vi "Update Component ID.vi"(8 "error in (no error)":errorcluster, 11 "SMO in":refnum<class "SMO.lvclass">) -> (0 "error out":errorcluster, 3 "SMO out":refnum<class "SMO.lvclass">)   [LabVIEW 2013, in "SMO.lvclass"]
uses:
  SMO.lvclass
  Support/Attribute.Identity/Attribute.Identity.lvclass
  Support/Attribute.Identity/Attribute.Identity.lvclass/Attribute.Identity.ctl
  Support/Attribute.Identity/Calculate Component ID.vi
  <vilib>/Utility/MD5Checksum.llb/MD5Checksum string.vi
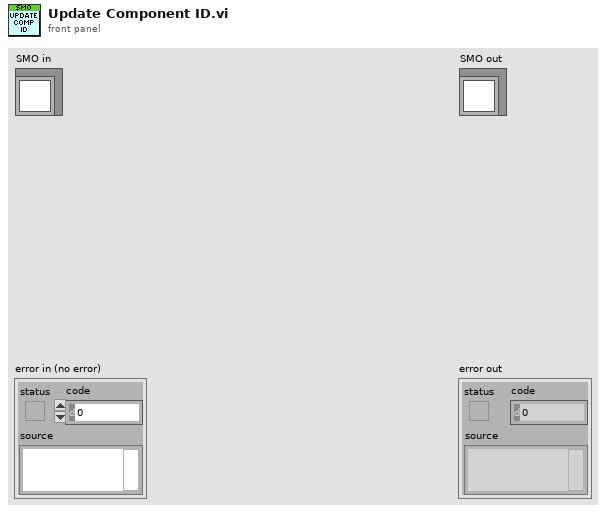
[diagram p1: front panel]
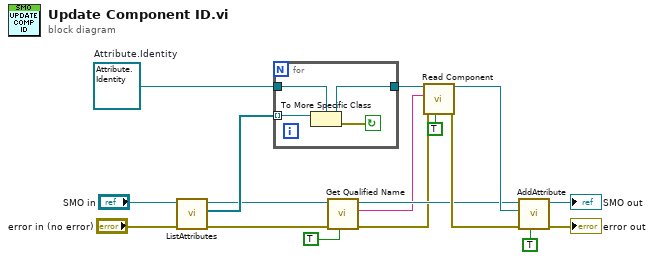
[diagram p0: block diagram]
diagram:
  w14 = refnum<class "Attribute.Identity.lvclass"> refnum  # Attribute.Identity
  n1 = call "ListAttributes.vi"("error in (no error)"="error in (no error)", "SMO in"="SMO in") -> ("error out"=w4:errorcluster, "[Attributes]"=w15:refnum<class "Attribute.lvclass">[], "SMO out"=w6:refnum<class "SMO.lvclass">)  [unwired: 7 in]
  n2 = for {
    tunnel: w15 -> [w21] mode=indexing
    tunnel: w14 -> [w20]
    tunnel: [w18] -> w13
    stop <- w19 continue-if-true
    n3 = To More Specific Class(target class=w20, reference=w21) -> (specific class reference=w18:refnum<class "Attribute.Identity.lvclass">, error out=w19:errorcluster)  [unwired: 1 in]
  }
  n4 = call "Get Qualified Name.vi"("Path? (F)"=TRUE, "error in (no error)"=w4, "SMO"=w6) -> ("error out"=w3:errorcluster, "Qualified Name"=w1:string, "SMO out"=w5:refnum<class "SMO.lvclass">)  [unwired: 6 in]
  n5 = call "Read Component.vi"("Create if non-existent? (F)"=TRUE, "error in (no error)"=w3, "Qualified Path"=w1, "Attribute.Identity in"=w13) -> ("error out"=w7:errorcluster, "Attribute.Identity out"=w9:refnum<class "Attribute.Identity.lvclass">)  [unwired: 5 in, 1 out]
  n6 = call "AddAttribute.vi"("Overwrite? (F)"=TRUE, "error in (no error)"=w7, "Attribute"=w9, "SMO in"=w5) -> ("error out"=→"error out":errorcluster, "SMO out"=→"SMO out":refnum<class "SMO.lvclass">)  [unwired: 6 in]
